vi "initiate.vi"(0 "reference in":refnum<class "excelFile.lvclass">, 5 "error in (no error)":errorcluster) -> (14 "reference out":refnum<class "excelFile.lvclass">, 19 "error out":errorcluster)   [LabVIEW 2015, in "excelFile.lvclass"]
uses:
  excelFile.lvclass
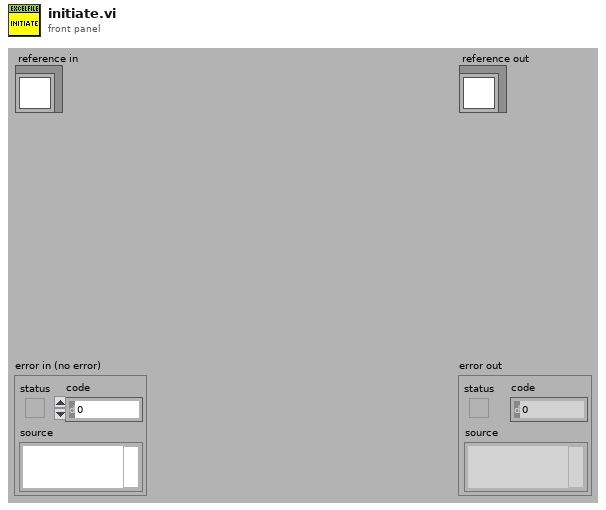
[diagram p1: front panel]
types:
  T1 = typedef "excelFile.lvclass/ObjectAttributesRef.ctl" = refnum<data-value>
  T2 = typedef "excelFile.lvclass/ObjectAttributes.ctl" = cluster{"MyAttribute":dbl, "path":string, "Refnum Excel":cluster{"Excel._Application":refnum<k7>, "Workbooks":refnum<k7>, "Open":refnum<k7>}, "data":string[][][], "fileType":T3, "sheetName":string[]}
  T3 = typedef "excelFile.lvclass/fileType.ctl" = enum16{"database", "CosmedTest"}
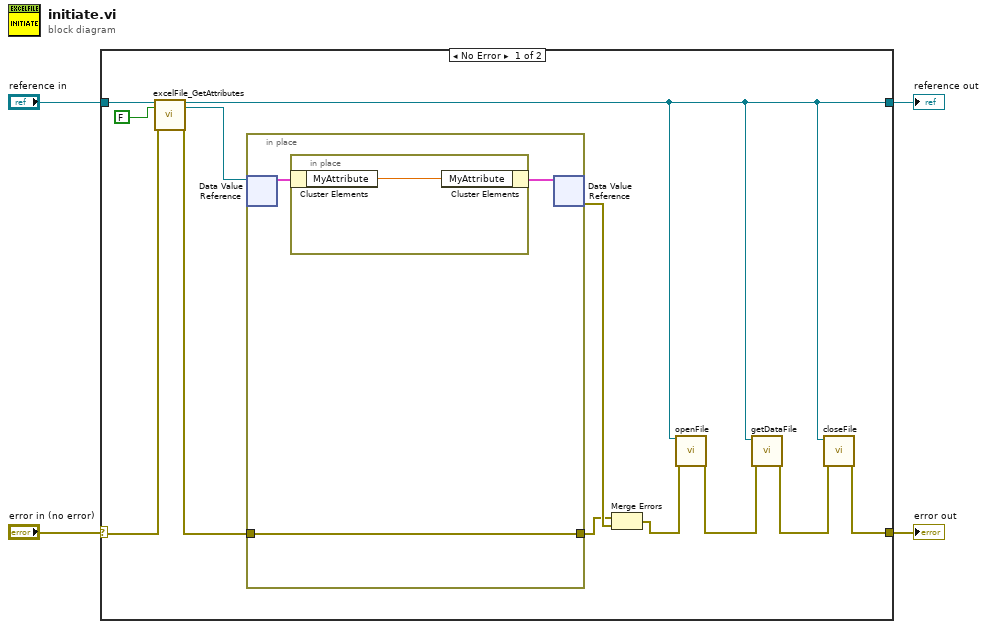
[diagram p0: block diagram]
diagram:
  n1 = case shown="No Error" "error in (no error)" {
    selector: "error in (no error)" -> [w12 w22]
    tunnel: [w6 w22] -> w3
    tunnel: [w5 w21] -> w1
    tunnel: "reference in" -> [w14 w21]
    frame No Error {
      n2 = call "excelFile_GetAttributes.vi"("reference in"=w14, "return data? (T)"=FALSE, "error in (no error)"=w12) -> ("reference out"=w5:refnum<class "excelFile.lvclass">, "attributes ref"=w10:T1, "error out"=w11:errorcluster)  [unwired: 13 in, 1 out]
      n3 = in-place {
        in-place-border: w11 -> [w17]
        in-place-border: [w17] -> w15
        n4 = in-place-dvr #1(w10) -> (w18:T2)  [unwired: 1 out]
        n5 = in-place {
          n6 = in-place-cluster #2(w18) -> ("MyAttribute"=w20:dbl)
          n7 = in-place-cluster #2("MyAttribute"=w20) -> (w19:T2)
        }
        n8 = in-place-dvr #1(w19) -> (w16:errorcluster)  [unwired: 1 out]
      }
      n9 = Merge Errors(w15, w16) -> (w9:errorcluster)
      n10 = call "openFile.vi"("reference in"=w5, "error in (no error)"=w9) -> ("error out"=w8:errorcluster)  [unwired: 16 in, 1 out]
      n11 = call "getDataFile.vi"("error in (no error)"=w8, "reference in"=w5) -> ("error out"=w7:errorcluster)  [unwired: 8 in, 1 out]
      n12 = call "closeFile.vi"("error in (no error)"=w7, "reference in"=w5) -> ("error out"=w6:errorcluster)  [unwired: 8 in, 1 out]
    }
    frame Error {
    }
  }
  "error out" <- w3
  "reference out" <- w1
